vi "pc_peaks_in_range.vi"(1 "range (Percent)":dbl, 2 "center offset":dbl, 3 "fit coeff":T1) -> (0 "in range?":bool)   [LabVIEW 2018, in "Plots.lvclass"]
doc: "checked whether both peaks are really at the correct offsets (within a certain range 0.2 -> 20 percent)."
uses:
  Plots.lvclass
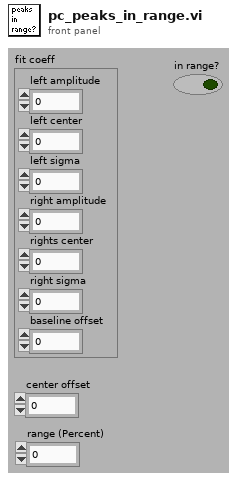
[diagram p1: front panel]
types:
  T1 = cluster{"left amplitude":dbl, "left center":dbl, "left sigma":dbl, "right amplitude":dbl, "rights center":dbl, "right sigma":dbl, "baseline offset":dbl}
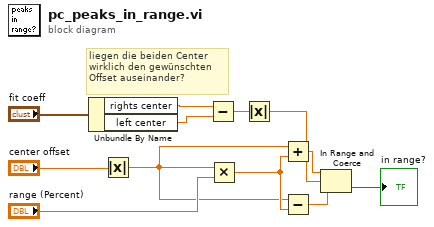
[diagram p0: block diagram]
diagram:
  # "liegen die beiden Center\nwirklich den gewünschten\nOffset auseinander?"
  n1 = Unbundle By Name("fit coeff") -> ("rights center"=w7:dbl, "left center"=w8:dbl)
  n2 = Absolute Value(x="center offset") -> (abs(x)=w3:dbl)
  n3 = Subtract(x=w7, y=w8) -> (x-y=w2:dbl)
  n4 = Multiply(x=w3, y="range (Percent)") -> (x*y=w11:dbl)
  n5 = Absolute Value(x=w2) -> (abs(x)=w1:dbl)
  n6 = Add(x=w3, y=w11) -> (x+y=w9:dbl)
  n7 = Subtract(x=w3, y=w11) -> (x-y=w10:dbl)
  n8 = In Range and Coerce(upper limit=w9, x=w1, lower limit=w10) -> (In Range?=→"in range?":bool)  [unwired: 1 out]
